vi "Auto Turn Precise.vi"(7 "Target Distance":dbl=90.0 format="%#_13g", 8 "Error In":errorcluster, 11 "Refnum's In":T1) -> (0 "Error Out":errorcluster, 3 "Refnum's Out":T1)   [LabVIEW 2016]
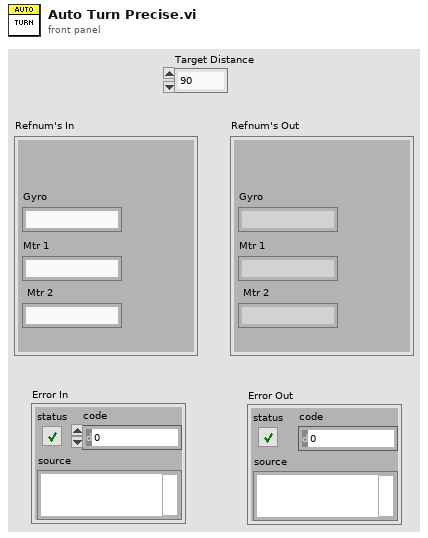
[diagram p1: front panel]
types:
  T1 = cluster{"Gyro":string, "Mtr 1":string, "Mtr 2":string}
  T2 = typedef "WPI_GyroDevRef.ctl" = cluster{"DevStatus":errorcluster, "Analog Channel":T3, "Offset":dbl, "Gain (VoltsPerDegree/Second)":dbl, "Gyro Type":enum16{"Analog", "XRS450"}, "Handle":i32, "SPI Bus":T4, "Device Found":bool, "Sample Rate":dbl, "Calibrate On Open":bool}
  T3 = typedef "FPGA_AIChannel.ctl" = enum8{"AI 0", "AI 1", "AI 2", "AI 3", "AI MXP 0", "AI MXP 1", "AI MXP 2", "AI MXP 3", "Invalid"}
  T4 = typedef "spi_bus.ctl" = enum16{"SPI On-Board, CS0", "SPI On-Board, CS1", "SPI On-Board, CS2", "SPI On-Board, CS3", "SPI MXP", "Invalid"}
  T5 = typedef "WPI_MotorControlDeviceRef.ctl" = cluster{"DeviceStatus":errorcluster, "Type":T6, "PWM":cluster{"PWM Channel":T7, "DeadBand":T8}, "CAN":cluster{"Device Number":u8, "SetOutput VI Ref":variant, "GetOutput VI Ref":variant, "Enable VI Ref":variant, "Disable VI Ref":variant, "Data":variant}, "Invert":bool}
  T6 = typedef "WPI_MotorControlType.ctl" = enum16{"PWM", "CAN"}
  T7 = typedef "FPGA_DIOPWMChannel.ctl" = enum8{"PWM 0", "PWM 1", "PWM 2", "PWM 3", "PWM 4", "PWM 5", "PWM 6", "PWM 7", "PWM 8", "PWM 9", "PWM MXP 0", "PWM MXP 1", "PWM MXP 2", "PWM MXP 3", "PWM MXP 4", "PWM MXP 5", "PWM MXP 6", "PWM MXP 7", "PWM MXP 8", "PWM MXP 9", "Invalid"}
  T8 = typedef "WPI_PWMDeadband.ctl" = cluster{"Name":string, "maxPositivePwm":i32, "minPositivePwm":i32, "centerPwm":i32, "maxNegativePwm":i32, "minNegativePwm":i32, "angularRange":u16}
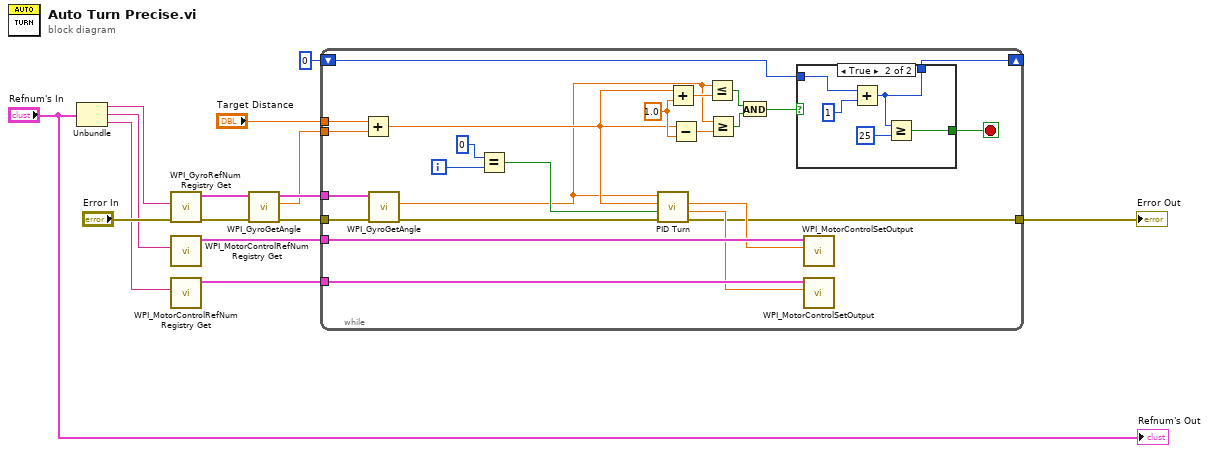
[diagram p0: block diagram]
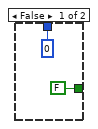
[diagram p2: hidden frame]
diagram:
  n1 = Unbundle("Refnum's In") -> ("Gyro"=w3:string, "Mtr 1"=w1:string, "Mtr 2"=w2:string)
  n2 = call <vilib>:"WPI_GyroRefNum Registry Get.vi"("error in (no error)"="Error In", "refnum name"=w3) -> ("error out"=w13:errorcluster, "GyroDevRef"=w14:T2)  [unwired: 8 in]
  n3 = call <vilib>:"WPI_MotorControlRefNum Registry Get.vi"("refnum name"=w1) -> ("MotorControlDevRef"=w6:T5)  [unwired: 9 in, 1 out]
  n4 = call <vilib>:"WPI_MotorControlRefNum Registry Get.vi"("refnum name"=w2) -> ("MotorControlDevRef"=w7:T5)  [unwired: 9 in, 1 out]
  n5 = call <vilib>:"WPI_GyroGetAngle.vi"("error in"=w13, "GyroDevRef"=w14) -> ("error out"=w9:errorcluster, "Angle"=w8:dbl, "GyroDevRef"=w10:T2)  [unwired: 5 in, 2 out]
  n6 = while {
    tunnel: w10 -> [w37]
    tunnel: w9 -> [w36]
    shift-right: [w29] -> _
    shift-left: 0 -> [w28]
    tunnel: "Target Distance" -> [w26]
    tunnel: w8 -> [w25]
    tunnel: w7 -> [w20]
    tunnel: w6 -> [w19]
    tunnel: [w16] -> w5
    i -> [w39]
    stop <- w21 stop-if-true
    w35 = 1.0 ("y")
    n7 = Add(x=w26, y=w25) -> (x+y=w24:dbl)
    n8 = call <vilib>:"WPI_GyroGetAngle.vi"("error in"=w36, "GyroDevRef"=w37) -> ("error out"=w23:errorcluster, "Angle"=w22:dbl)  [unwired: 5 in, 3 out]
    n9 = Equal?(x=0, y=w39) -> (x = y?=w27:bool)
    n10 = call "PID Turn.vi"("Error In"=w23, "Reinitialize"=w27, "Target Angle"=w24, "Gyro Angle"=w22) -> ("Error Out"=w16:errorcluster, "Right Power"=w17:dbl, "Left Power"=w18:dbl)  [unwired: 5 in]
    n11 = Add(x=w24, y=w35) -> (x+y=w34:dbl)
    n12 = Subtract(x=w24, y=w35) -> (x-y=w33:dbl)
    n13 = Less Or Equal?(x=w22, y=w34) -> (x <= y?=w32:bool)
    n14 = Greater Or Equal?(x=w22, y=w33) -> (x >= y?=w31:bool)
    n15 = And(x=w32, y=w31) -> (x .and. y?=w30:bool)
    n16 = case shown="True" w30 {
      tunnel: w28 -> [_ w45]
      tunnel: [0 w44] -> w29
      tunnel: [FALSE w42] -> w21
      frame False {
      }
      frame True {
        n17 = Add(x=w45, y=1) -> (x+y=w44:i32)
        n18 = Greater Or Equal?(x=w44, y=25) -> (x >= y?=w42:bool)
      }
    }
    n19 = call <vilib>:"WPI_MotorControlSetOutput.vi"("Output"=w18, "MotorControlDevRef"=w19) -> ()  [unwired: 7 in, 3 out]
    n20 = call <vilib>:"WPI_MotorControlSetOutput.vi"("Output"=w17, "MotorControlDevRef"=w20) -> ()  [unwired: 7 in, 3 out]
  }
  "Error Out" <- w5
  "Refnum's Out" <- "Refnum's In"
